vi "FMA1600A Device Units.vi"(8 "Error In":errorcluster, 10 "All Meter Data":T1, 11 "Meter":string) -> (0 "Error Out":errorcluster, 1 "Gas Temperature":string, 2 "Vol. Flow-Measured":string, 3 "Mass Flow-Measured":string, 4 "Gas Pressure":string, 5 "Gas Meter ID":string, 6 "Totalized Flow":string)   [LabVIEW 2018]
uses:
  Trunk/Range/Type Definitions/RANGE DAQ Data Four Meters.ctl
  Trunk/Range/Type Definitions/RANGE DAQ Data.ctl
  Type Definitions/FMA1600A Gas Type.ctl
  Type Definitions/FMA1600A Units String.ctl
  Trunk/Range/Type Definitions/RANGE GAS Data.ctl
  Trunk/Range/Type Definitions/RANGE Panel Data.ctl
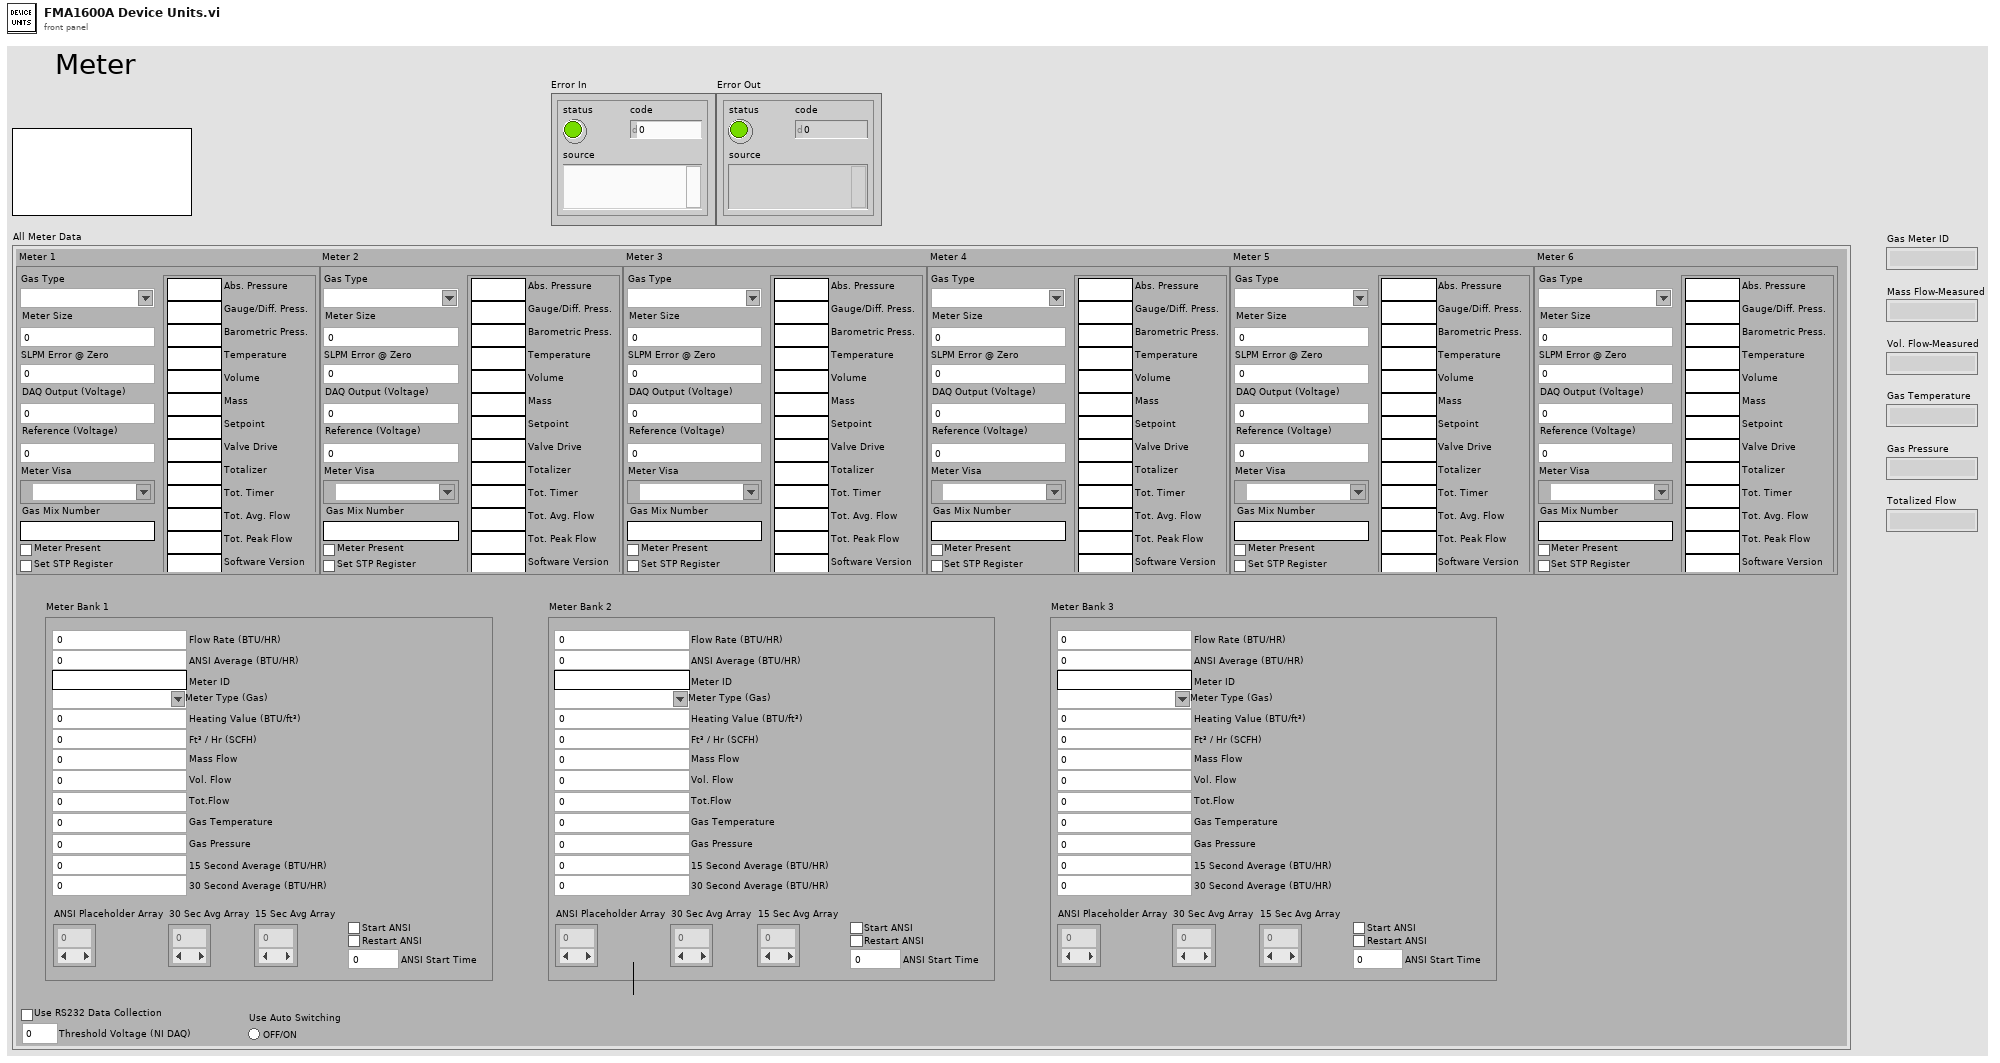
[diagram p1: front panel]
types:
  T1 = typedef "RANGE DAQ Data Four Meters.ctl" = cluster{"Meter 1":T2, "Meter 2":T2, "Meter 3":T2, "Meter 4":T2, "Meter 5":T2, "Meter 6":T2, "Meter Bank 1":T5, "Meter Bank 2":T5, "Meter Bank 3":T5, "Threshold Voltage (NI DAQ)":dbl, "Use RS232 Data Collection":bool, "Use Auto Switching":bool}
  T2 = typedef "RANGE DAQ Data.ctl" = cluster{"Meter Size":dbl, "DAQ Output (Voltage)":dbl, "Reference (Voltage)":dbl, "Meter Present":bool, "Meter Visa":refnum<visa-resource-name>, "Gas Type":T3, "SLPM Error @ Zero":dbl, "Gas Mix Number":string, "Set STP Register":bool, "Measurement Units":T4}
  T3 = typedef "FMA1600A Gas Type.ctl" = string
  T4 = typedef "FMA1600A Units String.ctl" = cluster{"Abs. Pressure":string, "Gauge/Diff. Press.":string, "Barometric Press.":string, "Temperature":string, "Volume":string, "Mass":string, "Setpoint":string, "Valve Drive":string, "Totalizer":string, "Tot. Timer":string, "Tot. Avg. Flow":string, "Tot. Peak Flow":string, "Software Version":string}
  T5 = typedef "RANGE GAS Data.ctl" = cluster{"Flow Rate (BTU/HR)":dbl, "ANSI Placeholder Array":dbl[], "15 Sec Avg Array":dbl[], "30 Sec Avg Array ":dbl[], "ANSI Average (BTU/HR)":dbl, "Panel Data":T6, "Start ANSI":bool, "ANSI Start Time":dbl, "Restart ANSI":bool, "Meter ID":string}
  T6 = typedef "RANGE Panel Data.ctl" = cluster{"Meter Type (Gas)":T3, "Heating Value (BTU/ft³)":dbl, "Ft³ / Hr (SCFH)":dbl, "15 Second Average (BTU/HR)":dbl, "30 Second Average (BTU/HR)":dbl, "Mass Flow":dbl, "Vol. Flow":dbl, "Gas Temperature":dbl, "Gas Pressure":dbl, "Tot.Flow":dbl}
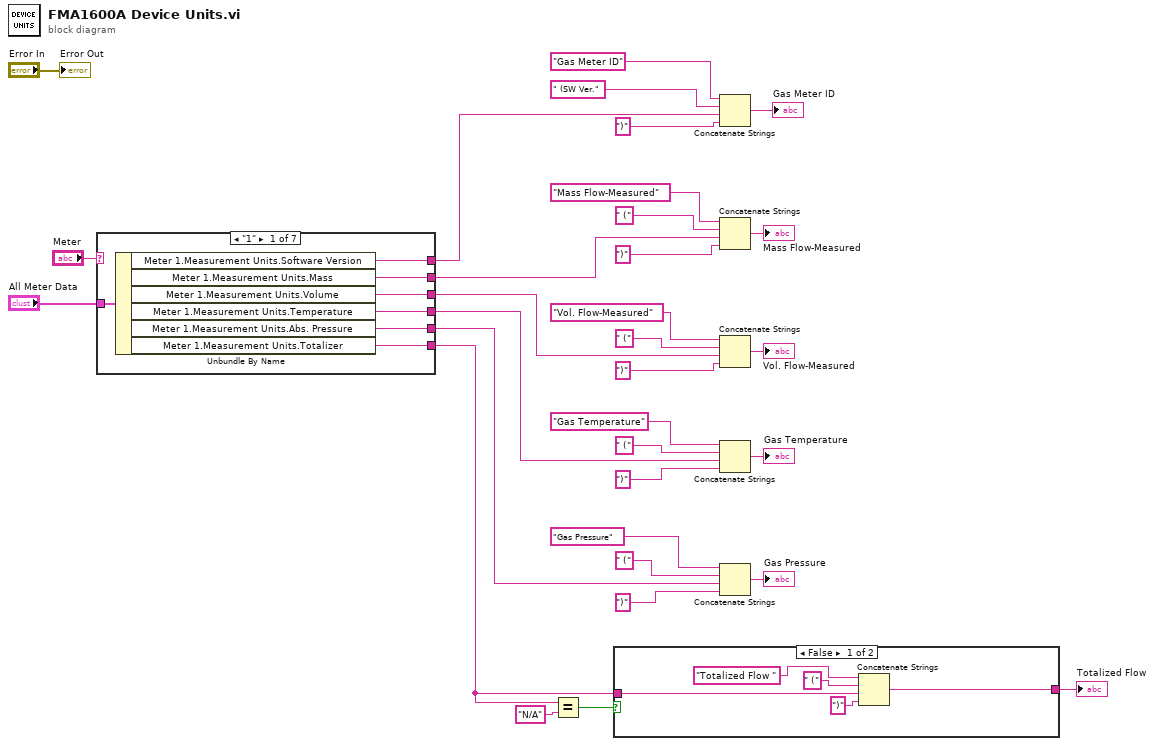
[diagram p0: block diagram]
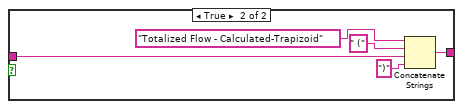
[diagram p2: hidden frame]
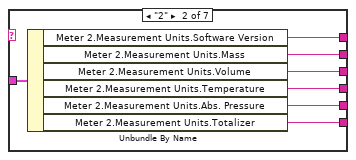
[diagram p3: hidden frame]
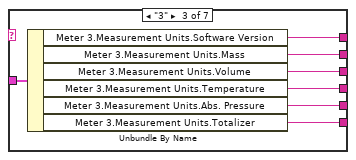
[diagram p4: hidden frame]
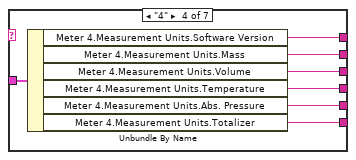
[diagram p5: hidden frame]
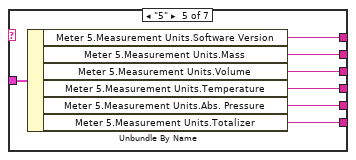
[diagram p6: hidden frame]
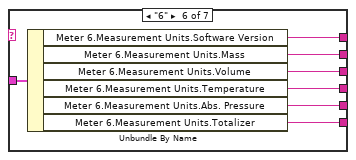
[diagram p7: hidden frame]
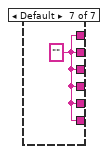
[diagram p8: hidden frame]
diagram:
  n1 = case shown="\"1\"" "Meter" {
    tunnel: [w39 w42 w49 w56 w63 w70 w75] -> w24
    tunnel: [w38 w43 w50 w57 w64 w71 w75] -> w5
    tunnel: [w37 w44 w51 w58 w65 w72 w75] -> w10
    tunnel: [w36 w45 w52 w59 w66 w73 w75] -> w13
    tunnel: [w35 w46 w53 w60 w67 w74 w75] -> w18
    tunnel: "All Meter Data" -> [w34 w41 w48 w55 w62 w69 _]
    tunnel: [w33 w40 w47 w54 w61 w68 w75] -> w31
    frame "1" {
      n2 = Unbundle By Name(w34) -> ("Meter 1.Measurement Units.Software Version"=w33:string, "Meter 1.Measurement Units.Mass"=w35:string, "Meter 1.Measurement Units.Volume"=w36:string, "Meter 1.Measurement Units.Temperature"=w37:string, "Meter 1.Measurement Units.Abs. Pressure"=w38:string, "Meter 1.Measurement Units.Totalizer"=w39:string)
    }
    frame "2" {
      n3 = Unbundle By Name(w41) -> ("Meter 2.Measurement Units.Software Version"=w40:string, "Meter 2.Measurement Units.Mass"=w46:string, "Meter 2.Measurement Units.Volume"=w45:string, "Meter 2.Measurement Units.Temperature"=w44:string, "Meter 2.Measurement Units.Abs. Pressure"=w43:string, "Meter 2.Measurement Units.Totalizer"=w42:string)
    }
    frame "3" {
      n4 = Unbundle By Name(w48) -> ("Meter 3.Measurement Units.Software Version"=w47:string, "Meter 3.Measurement Units.Mass"=w53:string, "Meter 3.Measurement Units.Volume"=w52:string, "Meter 3.Measurement Units.Temperature"=w51:string, "Meter 3.Measurement Units.Abs. Pressure"=w50:string, "Meter 3.Measurement Units.Totalizer"=w49:string)
    }
    frame "4" {
      n5 = Unbundle By Name(w55) -> ("Meter 4.Measurement Units.Software Version"=w54:string, "Meter 4.Measurement Units.Mass"=w60:string, "Meter 4.Measurement Units.Volume"=w59:string, "Meter 4.Measurement Units.Temperature"=w58:string, "Meter 4.Measurement Units.Abs. Pressure"=w57:string, "Meter 4.Measurement Units.Totalizer"=w56:string)
    }
    frame "5" {
      n6 = Unbundle By Name(w62) -> ("Meter 5.Measurement Units.Software Version"=w61:string, "Meter 5.Measurement Units.Mass"=w67:string, "Meter 5.Measurement Units.Volume"=w66:string, "Meter 5.Measurement Units.Temperature"=w65:string, "Meter 5.Measurement Units.Abs. Pressure"=w64:string, "Meter 5.Measurement Units.Totalizer"=w63:string)
    }
    frame "6" {
      n7 = Unbundle By Name(w69) -> ("Meter 6.Measurement Units.Software Version"=w68:string, "Meter 6.Measurement Units.Mass"=w74:string, "Meter 6.Measurement Units.Volume"=w73:string, "Meter 6.Measurement Units.Temperature"=w72:string, "Meter 6.Measurement Units.Abs. Pressure"=w71:string, "Meter 6.Measurement Units.Totalizer"=w70:string)
    }
    frame Default {
      w75 = "" ("Mass")
    }
  }
  n8 = Equal?(x=w24, y="N/A") -> (x = y?=w26:bool)
  n9 = case shown="False" w26 {
    tunnel: [w77 w84] -> w2
    tunnel: w24 -> [w76 w81]
    frame False {
      n10 = Concatenate Strings("Totalized Flow ", " (", w76, ")" ("string")) -> (w77:string)
    }
    frame True {
      n11 = Concatenate Strings("Totalized Flow - Calculated-Trapizoid", " (", w81, ")" ("string")) -> (w84:string)
    }
  }
  "Totalized Flow" <- w2
  n12 = Concatenate Strings("Gas Meter ID", " (SW Ver.", w31, ")" ("string")) -> (→"Gas Meter ID":string)
  n13 = Concatenate Strings("Mass Flow-Measured", " (", w18, ")" ("string")) -> (→"Mass Flow-Measured":string)
  n14 = Concatenate Strings("Vol. Flow-Measured", " (", w13, ")" ("string")) -> (→"Vol. Flow-Measured":string)
  n15 = Concatenate Strings("Gas Temperature", " (", w10, ")" ("string")) -> (→"Gas Temperature":string)
  n16 = Concatenate Strings("Gas Pressure", " (", w5, ")" ("string")) -> (→"Gas Pressure":string)
  "Error Out" <- "Error In"
